vi "Keithley_Write_1.vi"(1 "error in":errorcluster, 4 "C Max":dbl, 5 "C Min":dbl, 6 "PLC":u16, 7 "Num Pnts":dbl, 8 "VISA GPIB Resource 2":refnum<visa-resource-name>) -> (0 "error out":errorcluster, 3 "VISA GPIB Resource":refnum<visa-resource-name>)   [LabVIEW 2020]
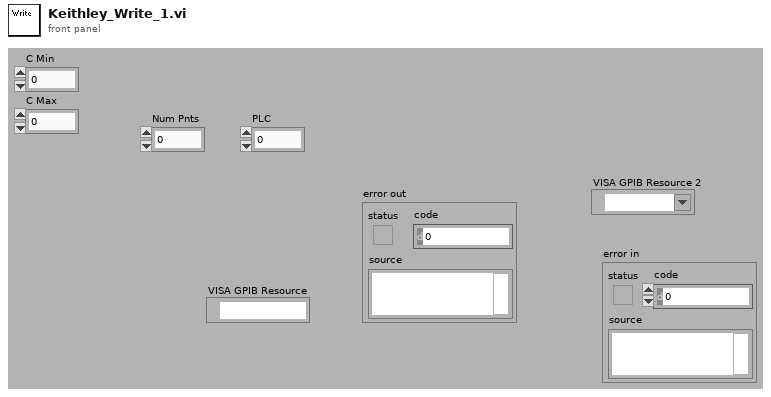
[diagram p1: front panel]
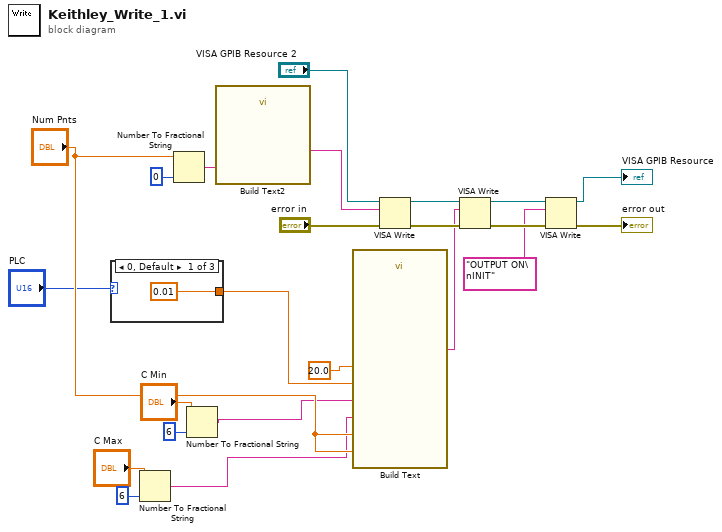
[diagram p0: block diagram]
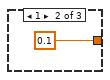
[diagram p2: hidden frame]
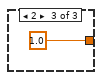
[diagram p3: hidden frame]
diagram:
  n1 = case shown="0, Default" "PLC" {
    tunnel: [0.01 0.1 1.0] -> w15
    frame 0, Default {
    }
    frame 1 {
    }
    frame 2 {
    }
  }
  n2 = Number To Fractional String(number="C Max", precision (6)=6) -> (F-format string=w8:string)  [unwired: 2 out]
  n3 = Number To Fractional String(number="Num Pnts", precision (6)=0) -> (F-format string=w23:string)  [unwired: 2 out]
  n4 = Number To Fractional String(number="C Min", precision (6)=6) -> (F-format string=w9:string)  [unwired: 2 out]
  n5 = call "Build Text2"("BUFF"=w23) -> ("Result"=w21:string)  [unwired: 3 in, 11 out]
  n6 = call "Build Text"("Cmax"=w8, "COUN"="Num Pnts", "Protection"=20.0, "PLC"=w15, "Cmin"=w9, "POINTS"="Num Pnts") -> ("Result"=w16:string)  [unwired: 3 in, 6 out]
  n7 = VISA Write(VISA resource name="VISA GPIB Resource 2", write buffer=w21, error in (no error)="error in") -> (VISA resource name out=w19:refnum<visa-resource-name>, error out=w20:errorcluster)  [unwired: 1 out]
  n8 = VISA Write(VISA resource name=w19, write buffer=w16, error in (no error)=w20) -> (VISA resource name out=w5:refnum<visa-resource-name>, error out=w4:errorcluster)  [unwired: 1 out]
  n9 = VISA Write(VISA resource name=w5, write buffer="OUTPUT ON\nINIT", error in (no error)=w4) -> (VISA resource name out=→"VISA GPIB Resource":refnum<visa-resource-name>, error out=→"error out":errorcluster)  [unwired: 1 out]
